vi "GetEvents.vi"(8 "error in (no error)":errorcluster, 11 "CameraTestingENI":refnum<class "CameraTestingENI.lvclass">) -> (0 "error out":errorcluster, 3 "CameraTestingENI":refnum<class "CameraTestingENI.lvclass">)   [LabVIEW 2020, in "CameraTestingProxy.lvlib" / "CameraTestingENI.lvclass"]
uses:
  CameraTestingENI.lvclass
  CameraTestingENI.lvclass/CameraTestingENI.ctl
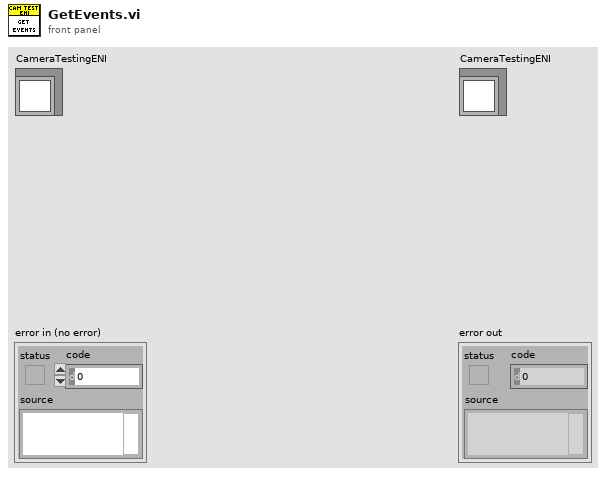
[diagram p1: front panel]
types:
  T1 = typedef "CameraTestingProxy.lvlib/CameraTestingENI.lvclass/RequestEventList.ctl" = cluster{"ConnectCmd":refnum<user-event>, "PlayCmd":refnum<user-event>, "SnapShoot":refnum<user-event>, "GetResolution":refnum<user-event>, "GetImageType":refnum<user-event>, "GetFrameRate":refnum<user-event>, "AcqVideoOptCodes":refnum<user-event>, "Quit":refnum<user-event>, "SetResolution":refnum<user-event>, "SetImageType":refnum<user-event>, "SetFrameRate":refnum<user-event>}
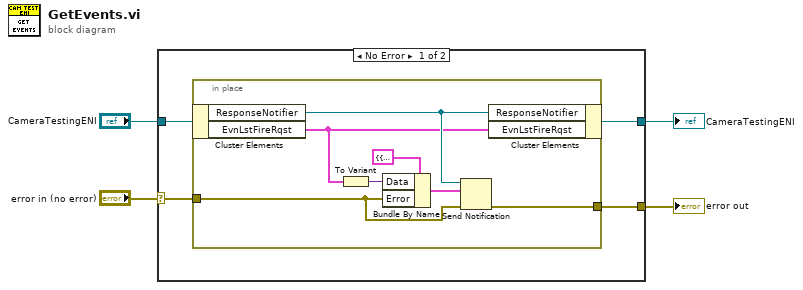
[diagram p0: block diagram]
diagram:
  n1 = case shown="No Error" "error in (no error)" {
    selector: "error in (no error)" -> [w7 w17]
    tunnel: [w6 w17] -> w3
    tunnel: [w5 w16] -> w1
    tunnel: "CameraTestingENI" -> [w8 w16]
    frame No Error {
      n2 = in-place {
        in-place-border: w7 -> [w11]
        in-place-border: [w12] -> w6
        n3 = in-place-cluster #1(w8) -> ("ResponseNotifier"=w10:refnum<notifier>, "EvnLstFireRqst"=w9:T1)
        n4 = To Variant(anything=w9) -> (Variant=w14:variant)
        n5 = Bundle By Name(cluster=cluster{"Error":errorcluster, "Data":variant} {"Error"={"status"=FALSE, "code"=0, "source"=""}, "Data"=variant} ("notification"), "Data"=w14, "Error"=w11) -> (w13:cluster{"Error":errorcluster, "Data":variant})
        n6 = Send Notification(notification=w13, notifier=w10, error in (no error)=w11) -> (error out=w12:errorcluster)  [unwired: 1 out]
        n7 = in-place-cluster #1("ResponseNotifier"=w10, "EvnLstFireRqst"=w9) -> (w5:refnum<class "CameraTestingENI.lvclass">)
      }
    }
    frame Error {
    }
  }
  "error out" <- w3
  "CameraTestingENI" <- w1
